vi "Lock-in auto sensitivity settings.vi"(4 "seconds to wait":u32, 5 "Voltage measure?":bool, 6 "Lower limit":dbl=10.0, 7 "Upper limit":dbl=90.0, 8 "error in (no error)":errorcluster, 9 "Check sensitivity":bool, 10 "Sensitivity in":dbl, 11 "VISA resource name":refnum<visa-resource-name>) -> (0 "error out":errorcluster, 1 "Data out":dbl, 2 "Sensitivity out":dbl)   [LabVIEW 2016]
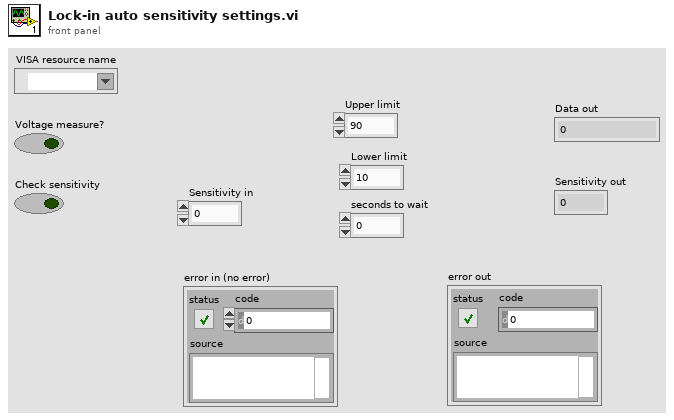
[diagram p1: front panel]
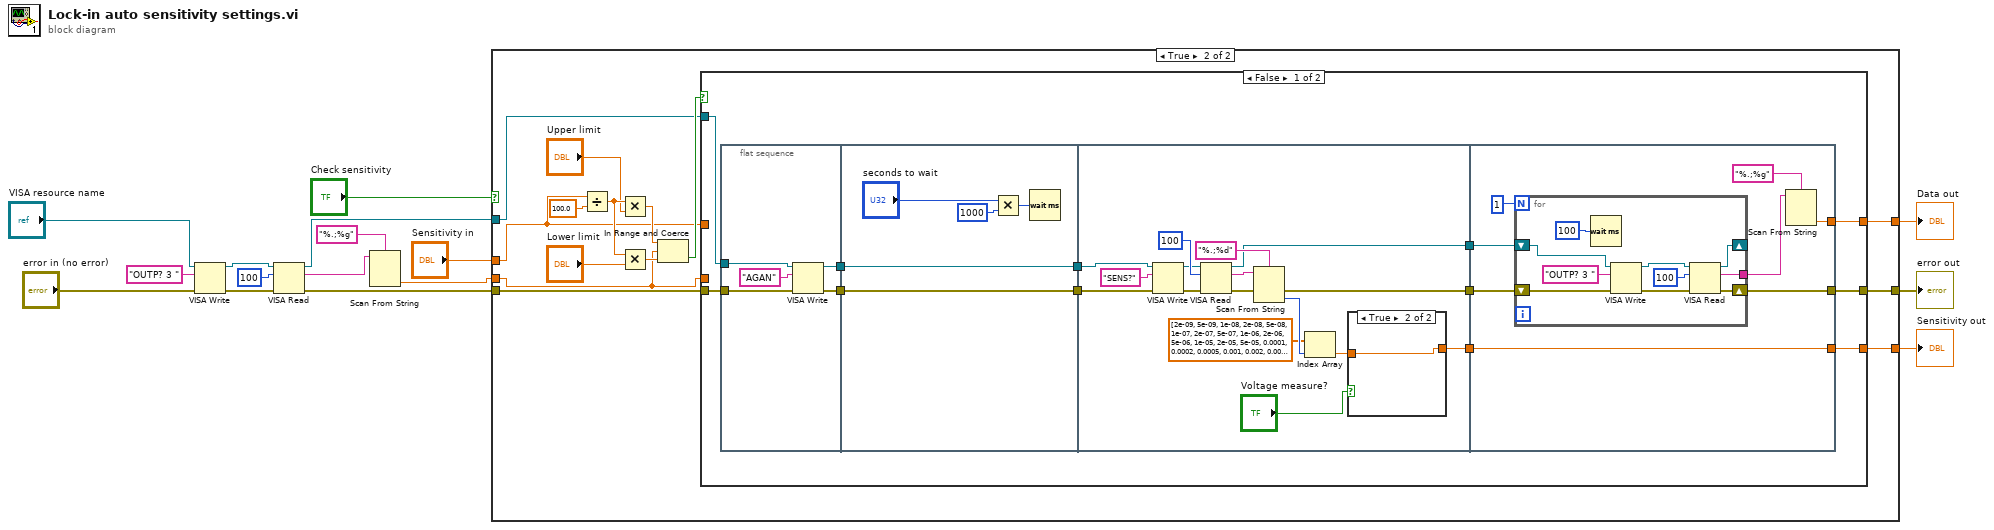
[diagram p0: block diagram]
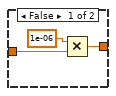
[diagram p3: hidden frame]
diagram:
  n1 = VISA Write(VISA resource name="VISA resource name", write buffer="OUTP? 3 " ("initial string"), error in (no error)="error in (no error)") -> (VISA resource name out=w15:refnum<visa-resource-name>, error out=w14:errorcluster)  [unwired: 1 out]
  n2 = VISA Read(VISA resource name=w15, byte count=u32 100, error in (no error)=w14) -> (VISA resource name out=w5:refnum<visa-resource-name>, read buffer=w12:string, error out=w4:errorcluster)  [unwired: 1 out]
  n3 = Scan From String(format string="%.;%g", input string=w12) -> (output 1=w7:dbl)  [unwired: 3 in, 3 out]
  n4 = case shown="True" "Check sensitivity" {
    tunnel: [w19 w26] -> w8
    tunnel: w7 -> [w19 w25]
    tunnel: w5 -> [_ w24]
    tunnel: w4 -> [w18 w23]
    tunnel: [w18 w22] -> w3
    tunnel: [w17 w21] -> w2
    tunnel: "Sensitivity in" -> [w17 w20]
    frame False {
    }
    frame True {
      n5 = Divide(x=w20, y=100.0) -> (x/y=w31:dbl)
      n6 = Multiply(x=w31, y="Upper limit") -> (x*y=w30:dbl)
      n7 = Multiply(x=w31, y="Lower limit") -> (x*y=w33:dbl)
      n8 = In Range and Coerce(upper limit=w30, x=w25, lower limit=w33) -> (In Range?=w27:bool)  [unwired: 1 out]
      n9 = case shown="False" w27 {
        tunnel: [w38 w96] -> w26
        tunnel: w25 -> [_ w96]
        tunnel: w24 -> [w45 _]
        tunnel: w23 -> [w42 w95]
        tunnel: [w39 w95] -> w22
        tunnel: [w37 w94] -> w21
        tunnel: w20 -> [_ w94]
        frame False {
          n10 = flat-sequence {
            tunnel: w45 -> [w49]
            tunnel: [w48] -> w43
            tunnel: w42 -> [w47]
            tunnel: [w46] -> w40
            tunnel: [w52] -> w44
            tunnel: w43 -> [w52]
            tunnel: [w51] -> w41
            tunnel: w40 -> [w51]
            tunnel: [w62] -> w36
            tunnel: [w57] -> w35
            tunnel: [w56] -> w34
            tunnel: w41 -> [w68]
            tunnel: w44 -> [w69]
            tunnel: [w83] -> w37
            tunnel: [w76] -> w38
            tunnel: [w77] -> w39
            tunnel: w36 -> [w79]
            tunnel: w35 -> [w83]
            tunnel: w34 -> [w78]
            frame #0 {
              n11 = VISA Write(VISA resource name=w49, write buffer="AGAN", error in (no error)=w47) -> (VISA resource name out=w48:refnum<visa-resource-name>, error out=w46:errorcluster)  [unwired: 1 out]
            }
            frame #1 {
              n12 = Multiply(x="seconds to wait", y=u32 1000) -> (x*y=w53:u32)
              n13 = Wait (ms)(milliseconds to wait=w53) -> ()  [unwired: 1 out]
            }
            frame #2 {
              n14 = VISA Write(VISA resource name=w69, write buffer="SENS?", error in (no error)=w68) -> (VISA resource name out=w67:refnum<visa-resource-name>, error out=w70:errorcluster)  [unwired: 1 out]
              n15 = VISA Read(VISA resource name=w67, byte count=u32 100, error in (no error)=w70) -> (VISA resource name out=w56:refnum<visa-resource-name>, read buffer=w64:string, error out=w63:errorcluster)  [unwired: 1 out]
              n16 = Scan From String(format string="%.;%d", input string=w64, error in=w63) -> (error out=w62:errorcluster, output 1=w65:i32)  [unwired: 2 in, 2 out]
              n17 = Index Array(array=dbl[] [2e-09, 5e-09, 1e-08, 2e-08, 5e-08, 1e-07, 2e-07, 5e-07, 1e-06, 2e-06, 5e-06, 1e-05, 2e-05, 5e-05, 0.0001, 0.0002, 0.0005, 0.001, 0.002, 0.005, 0.01, 0.02, 0.05, 0.1, 0.2, 0.5], index=w65) -> (element=w58:dbl)
              n18 = case shown="True" "Voltage measure?" {
                tunnel: [w72 w75] -> w57
                tunnel: w58 -> [w74 w75]
                frame False {
                  n19 = Multiply(x=1e-06, y=w74) -> (x*y=w72:dbl)
                }
                frame True {
                }
              }
            }
            frame #3 {
              n20 = for {
                N: 1 -> [_]
                tunnel: [w90] -> w81
                shift-right: [w85] -> _
                shift-left: w78 -> [w88]
                shift-right: [w86] -> w77
                shift-left: w79 -> [w87]
                n21 = Wait (ms)(milliseconds to wait=u32 100) -> ()  [unwired: 1 out]
                n22 = VISA Write(VISA resource name=w88, write buffer="OUTP? 3 " ("initial string"), error in (no error)=w87) -> (VISA resource name out=w92:refnum<visa-resource-name>, error out=w91:errorcluster)  [unwired: 1 out]
                n23 = VISA Read(VISA resource name=w92, byte count=u32 100, error in (no error)=w91) -> (VISA resource name out=w85:refnum<visa-resource-name>, read buffer=w90:string, error out=w86:errorcluster)  [unwired: 1 out]
              }
              n24 = Scan From String(format string="%.;%g", input string=w81) -> (output 1=w76:dbl)  [unwired: 3 in, 3 out]
            }
          }
        }
        frame True {
        }
      }
    }
  }
  "error out" <- w3
  "Data out" <- w8
  "Sensitivity out" <- w2
